vi "tag bus to profibus.vi"(10 "slave configuration":T2, 11 "data table in in":T1) -> (1 "Data":u8[](array[numeric]), 2 "slave index":i8, 3 "data table out":T1)   [LabVIEW 2013, in "Profibus Module runtime.lvclass"]
uses:
  Profibus Module runtime.lvclass
  profibus slave configuration.ctl
  profibus mapping configuration.ctl
  <vilib>/NI/Tag Bus/tag/Data Type.ctl
  <vilib>/NI/Tag Bus/table/data table.ctl
  <vilib>/NI/Tag Bus/table/data polymorphs/read one/read Double.vi
  <vilib>/NI/Tag Bus/table/data polymorphs/read one/read Single.vi
  <vilib>/NI/Tag Bus/table/data polymorphs/read one/read Boolean.vi
  <vilib>/NI/Tag Bus/table/data table.lvlib
  <vilib>/NI/Tag Bus/tag/tag descriptor.lvclass
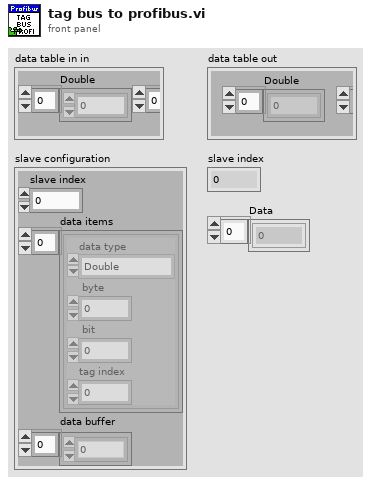
[diagram p1: front panel]
types:
  T1 = typedef "tag bus.lvlib/data table.lvlib/data table.ctl" = cluster{"Double":dbl[], "Single":sgl[], "I64":i64[], "I32":i32[], "I16":i16[], "I8":i8[], "U64":u64[], "U32":u32[], "U16":u16[], "U8":u8[], "Boolean":bool[], "String":string[], "Array of Double":cluster{"DBL Array":dbl[]}[], "Array of Single":cluster{"SGL Array":sgl[]}[], "Array of I64":cluster{"I64 Array":i64[]}[], "Array of I32":cluster{"I32 Array":i32[]}[], "Array of I16":cluster{"I16 Array":i16[]}[], "Array of I8":cluster{"I8 Array":i8[]}[], "Array of U64":cluster{"U64 Array":u64[]}[], "Array of U32":cluster{"U32 Array":u32[]}[], "Array of U16":cluster{"U16 Array":u16[]}[], "Array of U8":cluster{"U8 Array":u8[]}[], "Array of Boolean":cluster{"Boolean Array":bool[]}[], "Array of String":cluster{"String Array":string[]}[]}
  T2 = typedef "Profibus Module runtime.lvclass/profibus slave configuration.ctl" = cluster{"slave index":i8, "data items":T3[], "data buffer":u8[]}
  T3 = typedef "Profibus Module runtime.lvclass/profibus mapping configuration.ctl" = cluster{"data type":T4, " byte":i32, " bit":i32, "tag index":i32}
  T4 = typedef "tag bus.lvlib/tag descriptor.lvclass/Data Type.ctl" = enum16{"Double", "Single", "I64", "I32", "I16", "I8", "U64", "U32", "U16", "U8", "Boolean", "String", "Array of Double", "Array of Single", "Array of I64", "Array of I32", "Array of I16", "Array of I8", "Array of U64", "Array of U32", "Array of U16", "Array of U8", "Array of Boolean", "Array of String"}
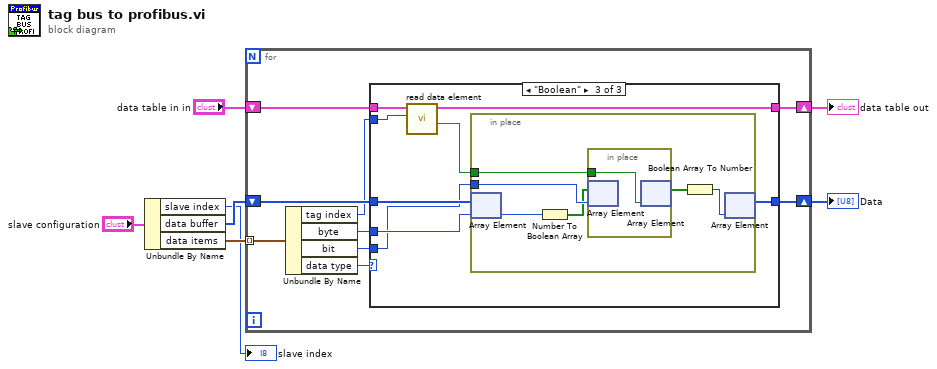
[diagram p0: block diagram]
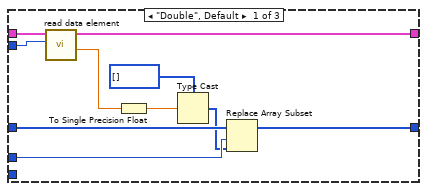
[diagram p2: hidden frame]
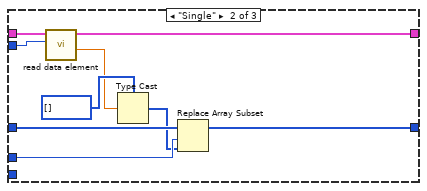
[diagram p3: hidden frame]
diagram:
  n1 = Unbundle By Name("slave configuration") -> ("slave index"=→"slave index":i8, "data buffer"=w6:u8[], "data items"=w4:T3[])
  n2 = for {
    tunnel: w4 -> [w16] mode=indexing
    shift-right: [w14] -> w5
    shift-left: w6 -> [w15]
    shift-right: [w9] -> w2
    shift-left: "data table in in" -> [w10]
    n3 = Unbundle By Name(w16) -> ("tag index"=w8:i32, "byte"=w13:i32, "bit"=w11:i32, "data type"=w12:T4)
    n4 = case shown="\"Boolean\"" w12 {
      tunnel: w8 -> [w18 w28 w36]
      tunnel: w15 -> [w24 w34 w43]
      tunnel: w13 -> [w22 w32 w42]
      tunnel: [w23 w33 w41] -> w14
      tunnel: w11 -> [_ _ w40]
      tunnel: w10 -> [w20 w30 w37]
      tunnel: [w19 w29 w38] -> w9
      frame "Double", Default {
        n5 = call-poly <vilib>:"read data element.vi"("index"=w18, "data table in"=w20) -> ("value"=w17:dbl, "data table out"=w19:T1)  [unwired: 8 in]
        n6 = To Single Precision Float(number=w17) -> (single precision float=w25:sgl)
        n7 = Type Cast(type=u8[] [] ("Array 2"), x=w25) -> (*(type *) &x=w21:u8[])
        n8 = Replace Array Subset(array=w24, new element=w21, index=w22) -> (w23:u8[])
      }
      frame "Single" {
        n9 = call-poly <vilib>:"read data element.vi"("index"=w28, "data table in"=w30) -> ("value"=w27:sgl, "data table out"=w29:T1)  [unwired: 8 in]
        n10 = Type Cast(type=u8[] [] ("Array 2"), x=w27) -> (*(type *) &x=w31:u8[])
        n11 = Replace Array Subset(array=w34, new element=w31, index=w32) -> (w33:u8[])
      }
      frame "Boolean" {
        n12 = call-poly <vilib>:"read data element.vi"("index"=w36, "data table in"=w37) -> ("value"=w39:bool, "data table out"=w38:T1)  [unwired: 8 in]
        n13 = in-place {
          in-place-border: w40 -> [w48]
          in-place-border: w39 -> [w47]
          n14 = in-place-array #1(w43, w42) -> (w49:u8)
          n15 = Number To Boolean Array(number=w49) -> (Boolean array=w44:bool[])
          n16 = in-place {
            in-place-border: w47 -> [w50]
            n17 = in-place-array #2(w44, w48) -> ()  [unwired: 1 out]
            n18 = in-place-array #2(w50) -> (w45:bool[])  [unwired: 1 out]
          }
          n19 = Boolean Array To Number(Boolean array=w45) -> (number=w46:u8)
          n20 = in-place-array #1(w46) -> (w41:u8[])  [unwired: 1 out]
        }
      }
    }
  }
  "Data" <- w5
  "data table out" <- w2
